vi "xy_to_xyz.vi"(2 "z":dbl, 3 "Position (2D)":cluster{dbl, dbl}) -> (0 "Position (3D)":cluster{dbl, dbl, dbl})   [LabVIEW 2019]
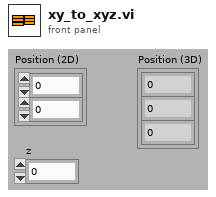
[diagram p1: front panel]
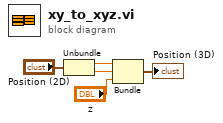
[diagram p0: block diagram]
diagram:
  n1 = Unbundle("Position (2D)") -> (w2:dbl, w3:dbl)
  n2 = Bundle(w2, w3, "z"="z") -> (→"Position (3D)":cluster{dbl, dbl, "z":dbl})  [unwired: 1 out]
